vi "Keithley 24XX Sweep and Acquire Measurements.vi"() -> ()   [LabVIEW 2024]
doc: "Configures a sweep and takes voltage and current readings at each point."
uses:
  <vilib>/Analysis/1siggen.llb/Ramp Pattern by Delta.vi
  Keithley 24XX.lvlib
  <vilib>/Analysis/NI_AALPro.lvlib
  <vilib>/Analysis/NI_AALBase.lvlib
  C:/Users/Public/OneDrive/Desktop/Keithley_2450_2470_1_4_0_LV2015_NewReadme2_2450-LV2015-1.4.0/Keithley 2450/Keithley 2450.lvlib
panel:
  in  "num_Vb_meas":i32
  out "current voltage 2450":dbl=6.7979141 format="%0.4f"
  out "mean current measured 2450":dbl=1.7421272433999997e-09 format="%0.5e"
  out "standard deviation current measured 2450":dbl=1.0038305493714546e-08 format="%0.5e"
  in  "Current Compliance Limit (0.1) 2450":dbl=5e-08
  in  "VISA resource name 2450":refnum<visa-resource-name>="GPIB0::1::INSTR"
  in  "Loop?":bool
  in  "Vb step":i32
  in  "Vb end":i32
  in  "Vb start":i32
  out "intercept":dbl
  out "slope":dbl
  out "Best Linear Fit":dbl[](array[numeric])
  out "XY Graph":T1(graph)
  in  "Source Mode  (0: Voltage)":u16(ring) items=["Voltage", "Current"]
  in  "Serial Configuration":T2={"Baud Rate"=9600, "Parity"=0, "Data Bits"=8, "Stop Bits"=10, "Flow Control"=0} {"Flow Control" items=["None", "XON/XOFF", "RTS/CTS", "XON/XOFF & RTS/CTS", "DTR/DSR", "XON/XOFF & DTR/DSR"]; "Stop Bits" items=["1.0"=10, "1.5"=15, "2.0"=20]; "Data Bits" items=["7"=7, "8"=8]; "Parity" items=["None", "Odd", "Even", "Mark", "Space"]; "Baud Rate" items=["300"=300, "600"=600, "1200"=1200, "2400"=2400, "4800"=4800, "9600"=9600, "19200"=19200]}
  in  "VISA resource name":refnum<visa-resource-name>
  in  "Timeout (10000 ms)":i32=10000 format="%#.6g"
  in  "Maximum Amplitude (2)":dbl=2.0
  in  "Minimum Amplitude (1)":dbl=1.0
  in  "Number of Points (5)":u32=5
  in  "Compliance  Level (0.1)":dbl=0.1
  # "(c) 2006 - 2015 National Instruments.  ALL RIGHTS RESERVED."
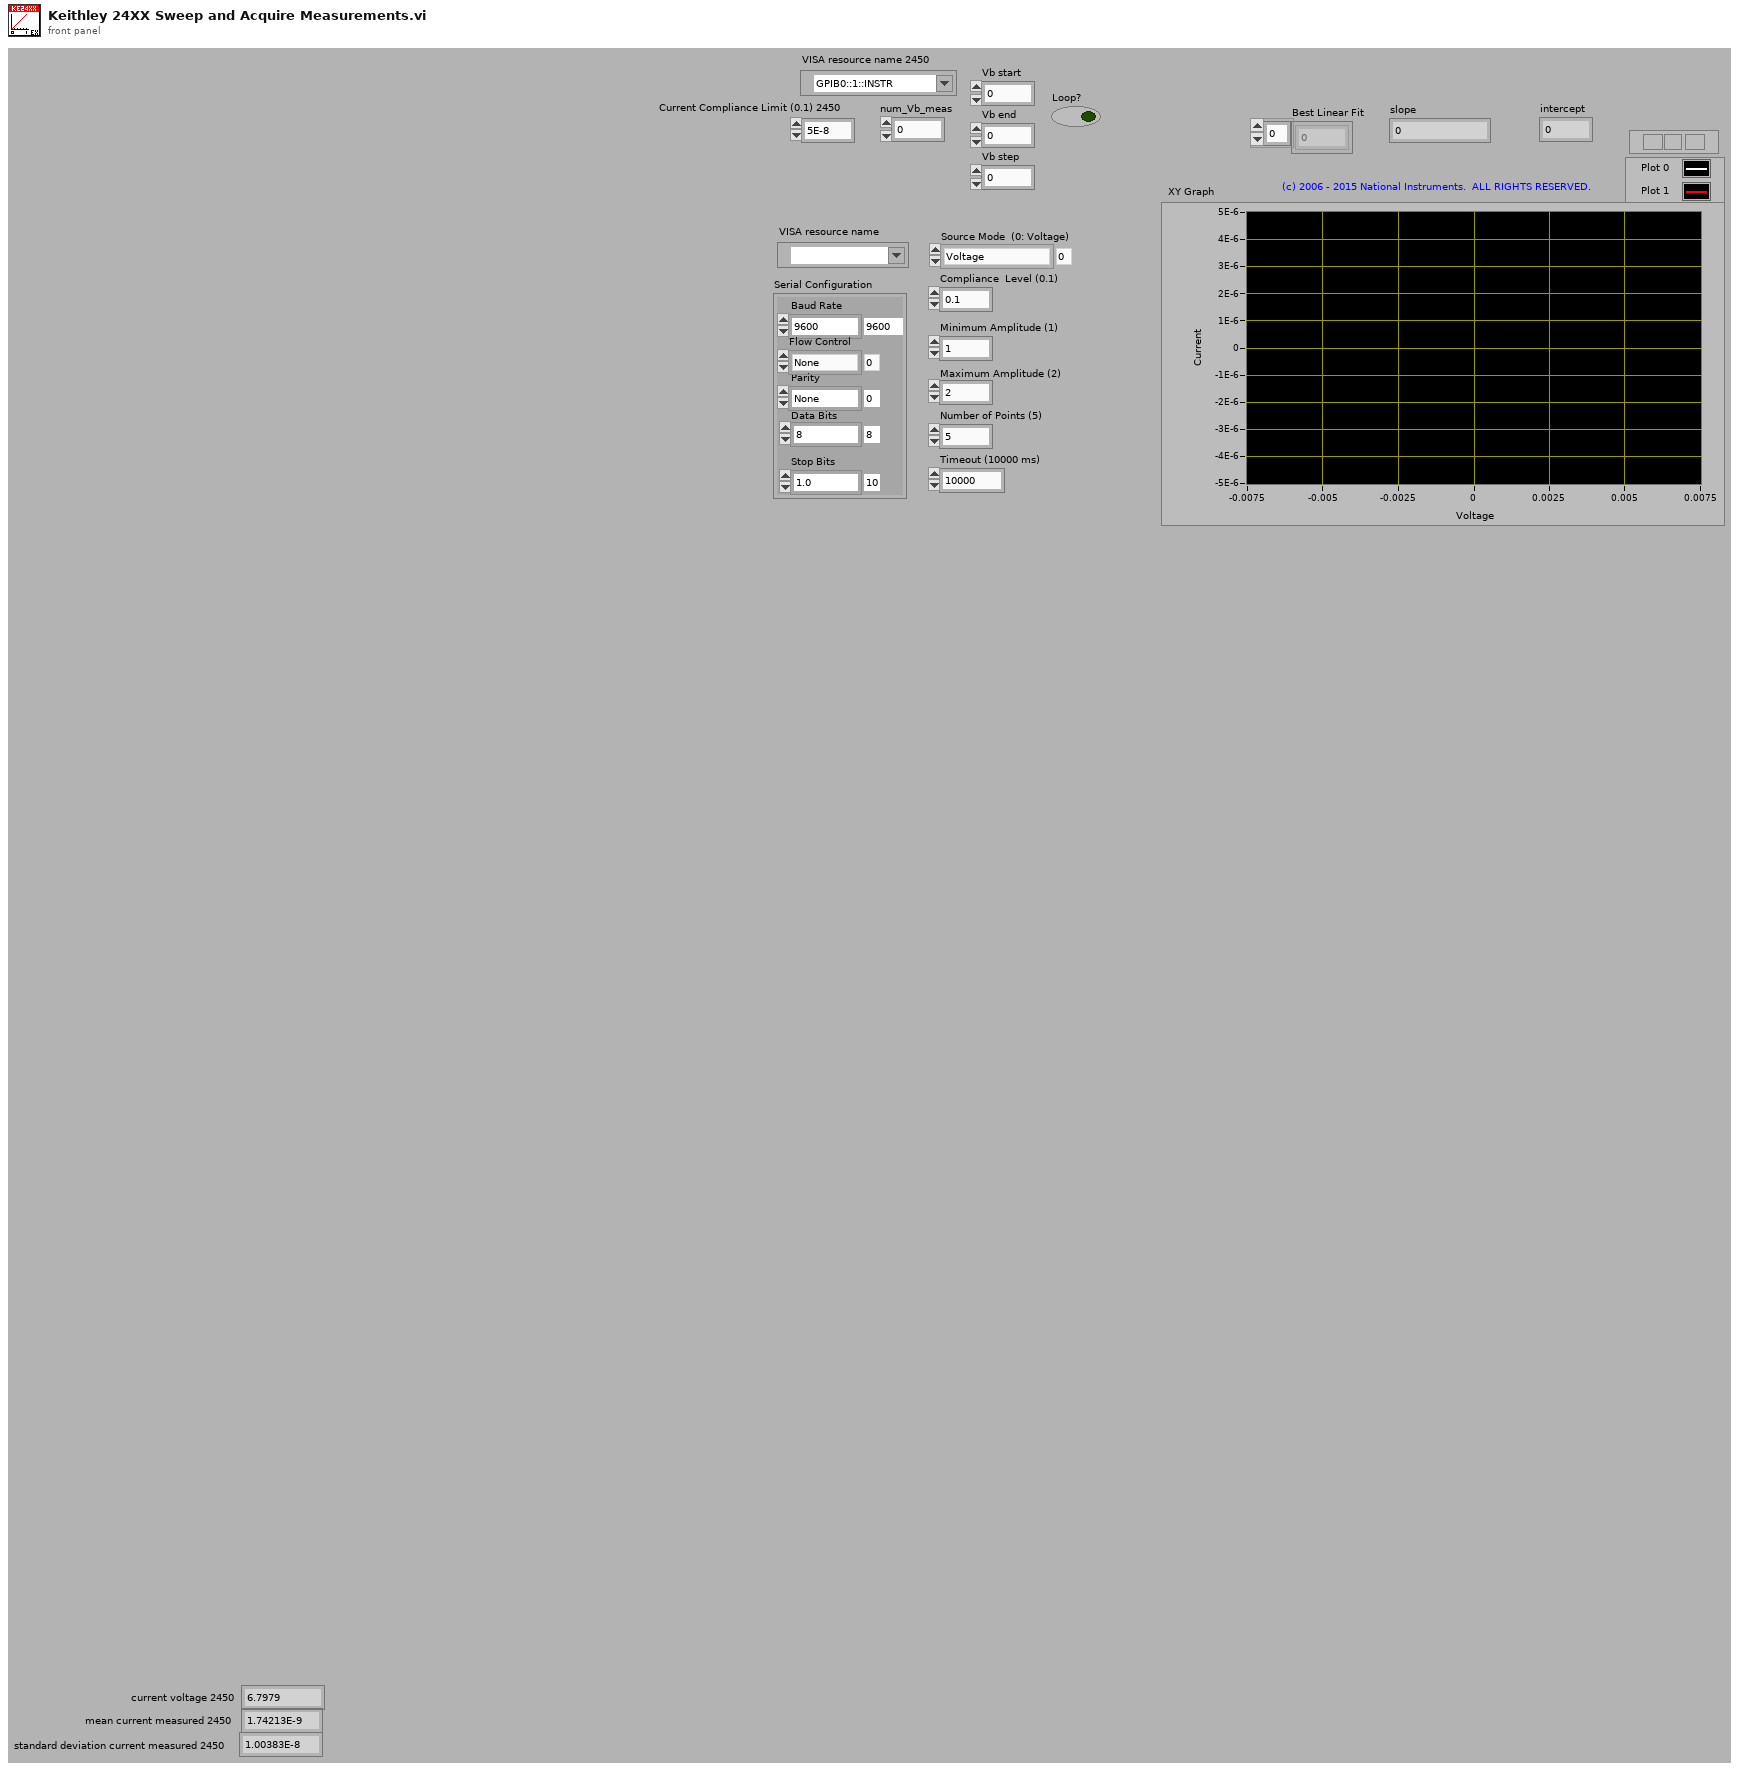
[diagram p1: front panel]
types:
  T1 = cluster{"Best Linear Fit":dbl[], "Current":sgl[]}[]
  T2 = cluster{"Baud Rate":u32, "Parity":u16, "Data Bits":u16, "Stop Bits":u16, "Flow Control":u16}
  T3 = cluster{"Best Linear Fit":dbl[], "Current":sgl[]}
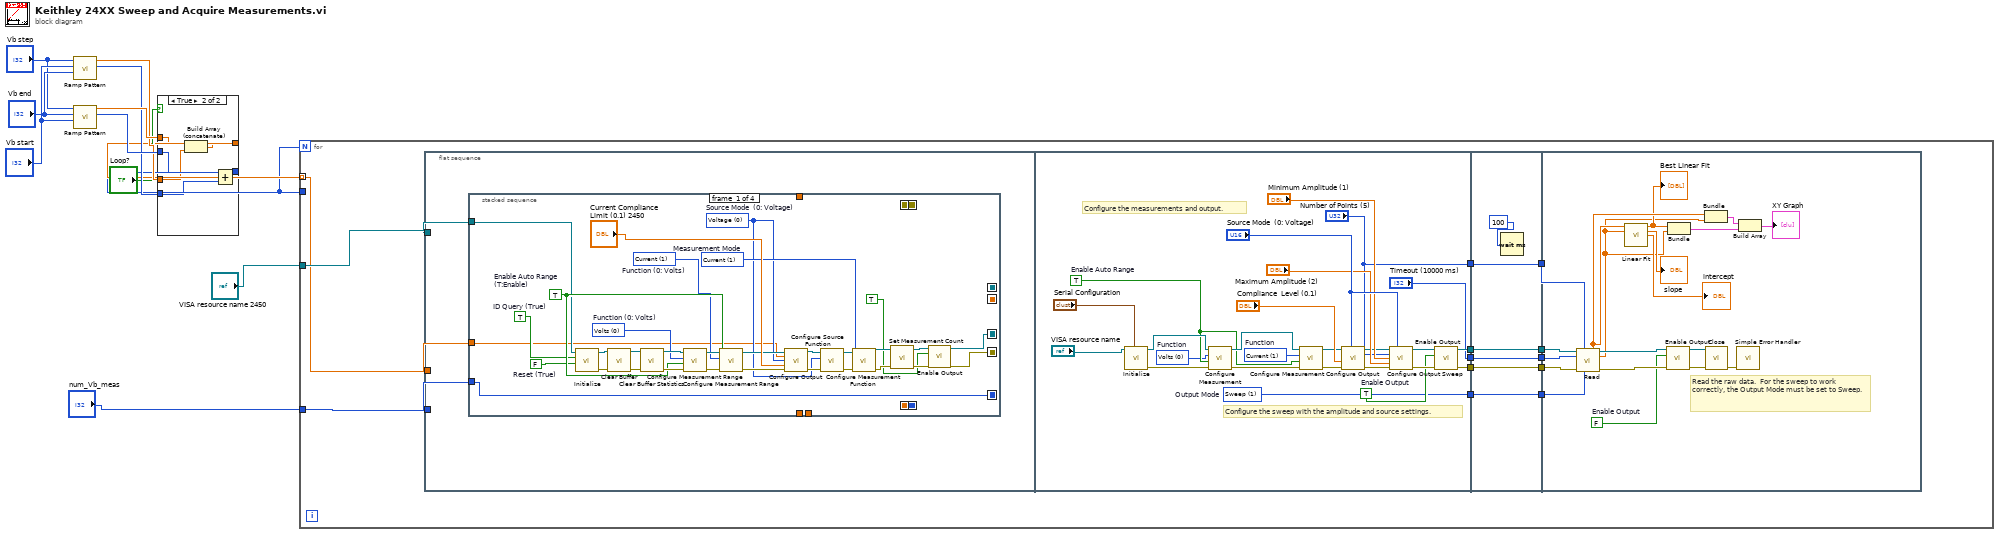
[diagram p0: block diagram]
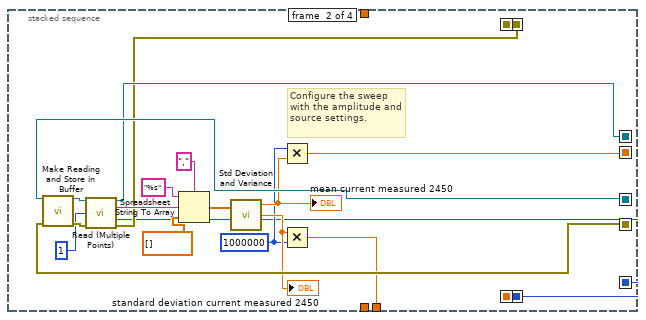
[diagram p3: hidden frame]
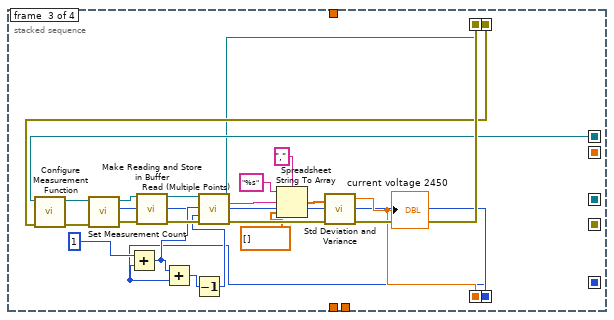
[diagram p4: hidden frame]
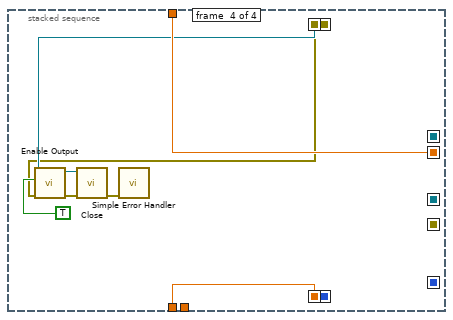
[diagram p5: hidden frame]
diagram:
  n1 = call-poly <vilib>:"Ramp Pattern.vi"("start"="Vb end", "end"="Vb start", "delta"="Vb step") -> ("samples"=w7:i32, "Ramp Pattern"=w6:dbl[])  [unwired: 6 in, 1 out]
  n2 = call-poly <vilib>:"Ramp Pattern.vi"("start"="Vb start", "end"="Vb end", "delta"="Vb step") -> ("samples"=w8:i32, "Ramp Pattern"=w9:dbl[])  [unwired: 6 in, 1 out]
  n3 = case shown="True" "Loop?" {
    tunnel: w9 -> [w14 w20]
    tunnel: w8 -> [w13 w17]
    tunnel: w7 -> [_ w15]
    tunnel: w6 -> [_ w19]
    tunnel: [w14 w18] -> w4
    tunnel: [w13 w16] -> w1
    frame False {
    }
    frame True {
      n4 = Build Array (concatenate)(w20, w19) -> (w18:dbl[])
      n5 = Add(x=w17, y=w15) -> (x+y=w16:i32)
    }
  }
  n6 = for {
    N: w1 -> [_]
    tunnel: w4 -> [w22] mode=indexing
    tunnel: w1 -> [_]
    tunnel: "VISA resource name 2450" -> [w23]
    tunnel: "num_Vb_meas" -> [w21]
    n7 = flat-sequence {
      tunnel: w23 -> [w36]
      tunnel: w22 -> [w35]
      tunnel: w21 -> [w34]
      tunnel: [w122] -> w33
      tunnel: ["Number of Points (5)"] -> w32
      tunnel: ["Timeout (10000 ms)"] -> w31
      tunnel: [w119] -> w30
      tunnel: [w118] -> w29
      tunnel: w33 -> [w148]
      tunnel: [w148] -> w28
      tunnel: w32 -> [w147]
      tunnel: [w147] -> w27
      tunnel: w31 -> [w146]
      tunnel: [w146] -> w26
      tunnel: w30 -> [w145]
      tunnel: [w145] -> w25
      tunnel: w29 -> [w144]
      tunnel: [w144] -> w24
      tunnel: w28 -> [w153]
      tunnel: w27 -> [w152]
      tunnel: w26 -> [w151]
      tunnel: w25 -> [w150]
      tunnel: w24 -> [w149]
      frame #0 {
        n8 = stacked-sequence {
          seq-local: [w41 _ _ _] -> [_ w86 _ _]
          seq-local: [w40 _ _ _] -> [_ w75 _ _]
          seq-local: [w37 _ _ _] -> [_ w69 _ _]
          seq-local: [_ w78 _ _] -> [_ _ w102 _]
          seq-local: [_ w77 _ _] -> [_ _ w103 _]
          seq-local: [_ w72 _ _] -> [_ _ w87 _]
          seq-local: [_ w69 _ _] -> [_ _ w89 _]
          seq-local: [_ w69 _ _] -> [_ _ w88 _]
          seq-local: [_ _ w101 _] -> [_ _ _ w111]
          seq-local: [_ _ w104 _] -> [_ _ _ w110]
          seq-local: [_ _ w87 _] -> [_ _ _ w117]
          seq-local: [_ _ w90 _] -> [_ _ _ w116]
          tunnel: w36 -> [w39 _ _ _]
          tunnel: w35 -> [w38 _ _ _]
          tunnel: w34 -> [w37 _ _ _]
          tunnel: [_ w74 _ _] -> _
          tunnel: [_ _ _ w117] -> _
          tunnel: [_ _ _ w116] -> _
          frame #0 {
            w42 = FALSE  # Reset (True)
            w43 = TRUE  # ID Query (True)
            w44 = u16 0 items=["Voltage", "Current"]  # Source Mode  (0: Voltage)
            w45 = u16 1 items=["Volts", "Current", "Auto Resistance", "Manual Resistance", "Digitize Voltage", "Digitize Current"]  # Measurement Mode
            w48 = TRUE  # Enable Auto Range (T:Enable)
            w46 = u16 1 items=["Volts", "Current", "Resistance"]  # Function (0: Volts)
            w47 = u16 0 items=["Volts", "Current", "Resistance"]  # Function (0: Volts)
            n9 = call "Initialize.vi"("Reset (True)"=w42, "ID Query (True)"=w43, "VISA resource name"=w39) -> ("error out"=w57:errorcluster, "VISA resource name out"=w56:refnum<visa-resource-name>)  [unwired: 7 in]
            n10 = call "Clear Buffer.vi"("VISA resource name"=w56, "error in (no error)"=w57) -> ("VISA resource name out"=w58:refnum<visa-resource-name>, "error out"=w61:errorcluster)  [unwired: 12 in]
            n11 = call "Clear Buffer Statistics.vi"("VISA resource name"=w58, "error in (no error)"=w61) -> ("VISA resource name out"=w59:refnum<visa-resource-name>, "error out"=w60:errorcluster)  [unwired: 12 in]
            n12 = call "Configure Measurement Range.vi"("error in (no error)"=w60, "Enable Auto Range (T:Enable)"=w48, "Function (0: Volts)"=w47, "VISA resource name"=w59) -> ("error out"=w54:errorcluster, "VISA resource name out"=w55:refnum<visa-resource-name>)  [unwired: 6 in]
            n13 = call "Configure Measurement Range.vi"("error in (no error)"=w54, "Enable Auto Range (T:Enable)"=w48, "Function (0: Volts)"=w46, "VISA resource name"=w55) -> ("error out"=w65:errorcluster, "VISA resource name out"=w64:refnum<visa-resource-name>)  [unwired: 6 in]
            n14 = call "Configure Output.vi"("VISA resource name"=w64, "Source Level (0)"=w38, "Source Mode  (0: Voltage)"=w44, "Source Limit Level (0.1)"="Current Compliance Limit (0.1) 2450", "error in (no error)"=w65) -> ("VISA resource name out"=w53:refnum<visa-resource-name>, "error out"=w52:errorcluster)  [unwired: 9 in]
            n15 = call "Configure Source Function.vi"("error in (no error)"=w52, "Function (0: Volts)"=w44, "VISA resource name"=w53) -> ("error out"=w51:errorcluster, "VISA resource name out"=w50:refnum<visa-resource-name>)  [unwired: 7 in]
            n16 = call "Configure Measurement Function.vi"("error in (no error)"=w51, "Function (0: Volts)"=w45, "VISA resource name"=w50) -> ("error out"=w62:errorcluster, "VISA resource name out"=w63:refnum<visa-resource-name>)  [unwired: 7 in]
            n17 = call "Set Measurement Count.vi"("error in (no error)"=w62, "VISA resource name"=w63) -> ("error out"=w68:errorcluster, "VISA resource name out"=w67:refnum<visa-resource-name>)  [unwired: 8 in]
            n18 = call "Enable Output.vi"("error in (no error)"=w68, "Enable Output (T: Enable)"=TRUE, "VISA resource name"=w67) -> ("error out"=w40:errorcluster, "VISA resource name out"=w41:refnum<visa-resource-name>)  [unwired: 7 in]
          }
          frame #1 {
            w70 = 1000000 ("Timeout (10000 ms)")
            # "Configure the sweep with the amplitude and source settings."
            n19 = call "Make Reading and Store in Buffer.vi"("VISA resource name"=w86, "error in (no error)"=w75) -> ("VISA resource name out"=w84:refnum<visa-resource-name>, "error out"=w85:errorcluster)  [unwired: 12 in]
            n20 = call "Read (Multiple Points).vi"("VISA resource name"=w84, "Start Index (1)"=u32 1, "End Index (1)"=w69, "error in (no error)"=w85) -> ("VISA resource name out"=w78:refnum<visa-resource-name>, "Data out"=w79:string, "error out"=w77:errorcluster)  [unwired: 9 in]
            n21 = Spreadsheet String To Array(delimiter (Tab)=",", format string="%s", spreadsheet string=w79, array type (2D Dbl)=dbl[] []) -> (array=w76:dbl[])
            n22 = call <vilib>:"Std Deviation and Variance.vi"("X"=w76) -> ("mean"=w71:dbl, "standard deviation"=w73:dbl)  [unwired: 1 in, 1 out]
            "mean current measured 2450" <- w71
            "standard deviation current measured 2450" <- w73
            n23 = Multiply(x=w70, y=w71) -> (x*y=w72:dbl)
            n24 = Multiply(x=w73, y=w70) -> (x*y=w74:dbl)
          }
          frame #2 {
            n25 = call "Configure Measurement Function.vi"("error in (no error)"=w103, "VISA resource name"=w102) -> ("error out"=w105:errorcluster, "VISA resource name out"=w109:refnum<visa-resource-name>)  [unwired: 8 in]
            n26 = call "Set Measurement Count.vi"("error in (no error)"=w105, "Measurement Count"=w89, "VISA resource name"=w109) -> ("error out"=w106:errorcluster, "VISA resource name out"=w100:refnum<visa-resource-name>)  [unwired: 7 in]
            n27 = Add(x=u32 1 ("Start Index (1)"), y=w88) -> (x+y=w92:u32)
            n28 = call "Make Reading and Store in Buffer.vi"("VISA resource name"=w100, "error in (no error)"=w106) -> ("VISA resource name out"=w108:refnum<visa-resource-name>, "error out"=w107:errorcluster)  [unwired: 12 in]
            n29 = Add(x=w92, y=w88) -> (x+y=w93:u32)
            n30 = Decrement(x=w93) -> (x-1=w91:u32)
            n31 = call "Read (Multiple Points).vi"("VISA resource name"=w108, "Start Index (1)"=w92, "End Index (1)"=w91, "error in (no error)"=w107) -> ("VISA resource name out"=w101:refnum<visa-resource-name>, "Data out"=w96:string, "error out"=w104:errorcluster)  [unwired: 9 in]
            n32 = Spreadsheet String To Array(delimiter (Tab)=",", format string="%s", spreadsheet string=w96, array type (2D Dbl)=dbl[] []) -> (array=w95:dbl[])
            n33 = call <vilib>:"Std Deviation and Variance.vi"("X"=w95) -> ("mean"=w90:dbl)  [unwired: 1 in, 2 out]
            "current voltage 2450" <- w90
          }
          frame #3 {
            n34 = call "Enable Output.vi"("error in (no error)"=w110, "Enable Output (T: Enable)"=TRUE, "VISA resource name"=w111) -> ("error out"=w114:errorcluster, "VISA resource name out"=w113:refnum<visa-resource-name>)  [unwired: 7 in]
            n35 = call "Close.vi"("error in (no error)"=w114, "VISA resource name"=w113) -> ("error out"=w115:errorcluster)  [unwired: 9 in]
            n36 = call <vilib>:"Simple Error Handler.vi"("error in (no error)"=w115) -> ()  [unwired: 4 in, 5 out]
          }
        }
      }
      frame #1 {
        w126 = TRUE  # Enable Output
        w125 = TRUE  # Enable Auto Range
        w124 = u16 1 items=["Volts", "Current", "Resistance"]  # Function
        w123 = u16 0 items=["Volts", "Current", "Resistance"]  # Function
        w118 = u16 1 items=["Fixed", "Sweep", "List"]  # Output Mode
        # "Configure the sweep with the amplitude and source settings."
        # "Configure the measurements and output."
        n37 = call "Initialize.vi"("Serial Configuration"="Serial Configuration", "VISA resource name"="VISA resource name") -> ("error out"=w128:errorcluster, "VISA resource name out"=w127:refnum<visa-resource-name>)  [unwired: 8 in]
        n38 = call "Configure Measurement.vi"("error in (no error)"=w128, "Enable Auto Range (T:Enable)"=w125, "Function (0: Volts)"=w123, "VISA resource name"=w127) -> ("error out"=w129:errorcluster, "VISA resource name out"=w130:refnum<visa-resource-name>)  [unwired: 6 in]
        n39 = call "Configure Measurement.vi"("error in (no error)"=w129, "Enable Auto Range (T:Enable)"=w125, "Function (0: Volts)"=w124, "VISA resource name"=w130) -> ("error out"=w132:errorcluster, "VISA resource name out"=w131:refnum<visa-resource-name>)  [unwired: 6 in]
        n40 = call "Configure Output.vi"("Source Mode  (0: Voltage)"="Source Mode  (0: Voltage)", "error in (no error)"=w132, "Compliance  Level (0.1)"="Compliance  Level (0.1)", "VISA resource name"=w131) -> ("error out"=w133:errorcluster, "VISA resource name out"=w134:refnum<visa-resource-name>)  [unwired: 6 in]
        n41 = call "Configure Output Sweep.vi"("VISA resource name"=w134, "Source Mode  (0: Voltage)"="Source Mode  (0: Voltage)", "Number of Points (5)"="Number of Points (5)", "Minimum Amplitude (1)"="Minimum Amplitude (1)", "Maximum Amplitude (2)"="Maximum Amplitude (2)", "error in (no error)"=w133) -> ("VISA resource name out"=w139:refnum<visa-resource-name>, "error out"=w140:errorcluster)  [unwired: 8 in]
        n42 = call "Enable Output.vi"("error in (no error)"=w140, "Enable Output (T: Enable)"=w126, "VISA resource name"=w139) -> ("error out"=w119:errorcluster, "VISA resource name out"=w122:refnum<visa-resource-name>)  [unwired: 7 in]
      }
      frame #2 {
        n43 = Wait (ms)(milliseconds to wait=u32 100) -> ()  [unwired: 1 out]
      }
      frame #3 {
        w154 = FALSE  # Enable Output
        # "Read the raw data.  For the sweep to work correctly, the Output Mode must be set to Sweep."
        n44 = call-poly "Read.vi"("VISA resource name"=w153, "Sample Count (1)"=w152, "Timeout (10000 ms)"=w151, "error in (no error)"=w150, "Output Mode (0: Fixed)"=w149) -> ("Voltage"=w160:sgl[], "VISA resource name out"=w163:refnum<visa-resource-name>, "Current"=w158:sgl[], "error out"=w164:errorcluster)  [unwired: 4 in, 3 out]
        n45 = call <vilib>:"Linear Fit.vi"("Y"=w160, "X"=w158) -> ("Best Linear Fit"=w159:dbl[], "slope"=→"slope":dbl, "intercept"=→"intercept":dbl)  [unwired: 9 in, 2 out]
        "Best Linear Fit" <- w159
        n46 = call "Enable Output.vi"("error in (no error)"=w164, "Enable Output (T: Enable)"=w154, "VISA resource name"=w163) -> ("error out"=w165:errorcluster, "VISA resource name out"=w166:refnum<visa-resource-name>)  [unwired: 7 in]
        n47 = Bundle("Best Linear Fit"=w159, "Current"=w158) -> (w156:T3)  [unwired: 1 in]
        n48 = Bundle("Voltage"=w160, "Current"=w158) -> (w157:cluster{"Voltage":sgl[], "Current":sgl[]})  [unwired: 1 in]
        n49 = call "Close.vi"("error in (no error)"=w165, "VISA resource name"=w166) -> ("error out"=w167:errorcluster)  [unwired: 9 in]
        n50 = call <vilib>:"Simple Error Handler.vi"("error in (no error)"=w167) -> ()  [unwired: 4 in, 5 out]
        n51 = Build Array(w157, w156) -> (→"XY Graph":T1)
      }
    }
  }
